vi "Report Bool Command.vi"(7 "Level (Info)":T2=enum."Info", 8 "error in (no error)":errorcluster, 10 "Command":T1, 11 "Module in":refnum<class "Module.lvclass">) -> (0 "error out":errorcluster, 3 "Module out":refnum<class "Module.lvclass">)   [LabVIEW 2020, in "Volatus.lvlib" / "Module.lvclass"]
uses:
  Module.lvclass
  Event Level.ctl
  Module.lvclass/Module.ctl
  lv-vecto/Vecto/Vecto.lvlib
  Volatus.lvlib
  messages/CmdDigital/Data.ctl
  messages/CmdDigital/CmdDigital.lvlib
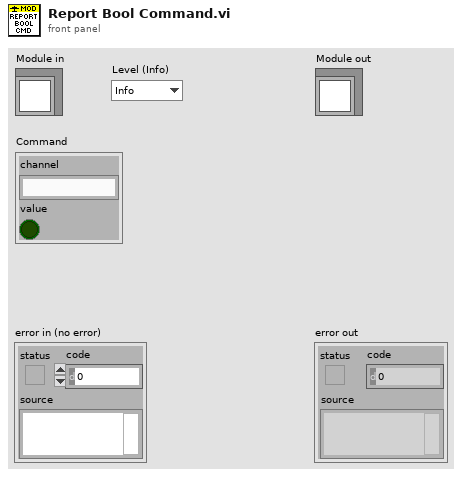
[diagram p1: front panel]
types:
  T1 = typedef "CmdDigital.lvlib/Data.ctl" = cluster{"channel":string, "value":bool}
  T2 = typedef "Volatus.lvlib/Event Level.ctl" = enum16{"Debug", "Info", "Warning", "Error"}
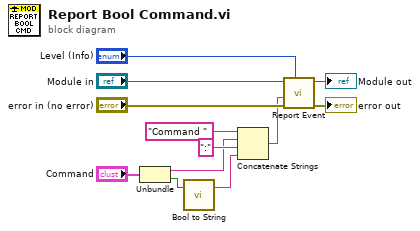
[diagram p0: block diagram]
diagram:
  n1 = Unbundle("Command") -> ("channel"=w2:string, "value"=w1:bool)
  n2 = call "Bool to String.vi"("Bool"=w1) -> ("String"=w6:string)  [unwired: 2 in]
  n3 = Concatenate Strings("Command " ("string"), w2, ":" ("string"), w6) -> (w5:string)
  n4 = call "Report Event.vi"("Level (Info)"="Level (Info)", "error in (no error)"="error in (no error)", "Message"=w5, "Module in"="Module in") -> ("error out"=→"error out":errorcluster, "Module out"=→"Module out":refnum<class "Module.lvclass">)  [unwired: 6 in]
